vi "LVJSON Tester.vi"() -> ()   [LabVIEW 2013]
panel:
  out "value":string
  out "error out":errorcluster
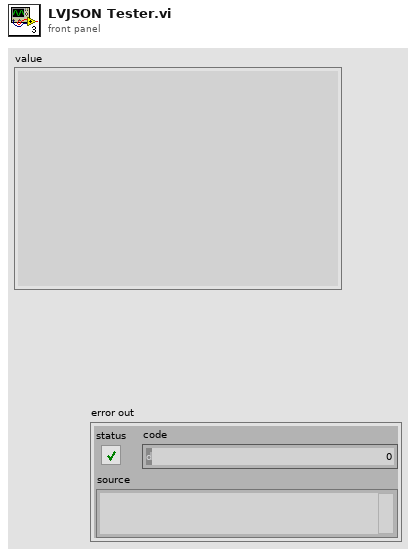
[diagram p1: front panel]
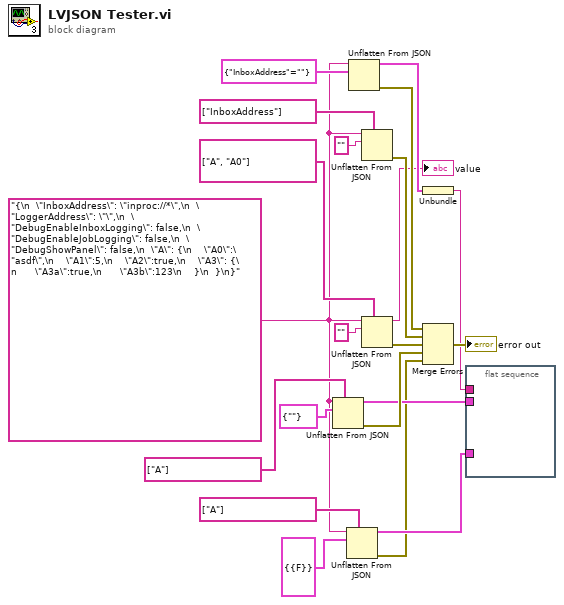
[diagram p0: block diagram]
diagram:
  w3 = "{\n  \"InboxAddress\": \"inproc://*\",\n  \"LoggerAddress\": \"\",\n  \"DebugEnableInboxLogging\": false,\n  \"DebugEnableJobLogging\": false,\n  \"DebugShowPanel\": false,\n  \"A\": {\n    \"A0\":\"asdf\",\n    \"A1\":5,\n    \"A2\":true,\n    \"A3\": {\n      \"A3a\":true,\n      \"A3b\":123\n    }\n  }\n}" ("Actor 1 Configuration")
  n1 = Unflatten From JSON(path=string[] ["A"], JSON string=w3, type and defaults=cluster{"A0":string} {"A0"=""}) -> (value=w7:cluster{"A0":string}, error out=w9:errorcluster)  [unwired: 4 in]
  n2 = Unflatten From JSON(path=string[] ["A"], JSON string=w3, type and defaults=cluster{"A3":cluster{"A3a":bool}} {"A3"={"A3a"=FALSE}}) -> (value=w2:cluster{"A3":cluster{"A3a":bool}}, error out=w1:errorcluster)  [unwired: 4 in]
  n3 = Unflatten From JSON(JSON string=w3, type and defaults=cluster{"InboxAddress":string} {"InboxAddress"=""}) -> (value=w20:cluster{"InboxAddress":string}, error out=w19:errorcluster)  [unwired: 5 in]
  n4 = Unflatten From JSON(path=string[] ["InboxAddress"], JSON string=w3, type and defaults="") -> (error out=w17:errorcluster)  [unwired: 4 in, 1 out]
  n5 = Unflatten From JSON(path=string[] ["A", "A0"], JSON string=w3, type and defaults="") -> (value=→"value":string, error out=w11:errorcluster)  [unwired: 4 in]
  n6 = Unbundle(w20) -> ("InboxAddress"=w6:string)
  n7 = Merge Errors(w19, w17, w11, w9, w1) -> (→"error out":errorcluster)
  n8 = flat-sequence {
    tunnel: w7 -> [_]
    tunnel: w6 -> [_]
    tunnel: w2 -> [_]
    frame #0 {
    }
  }
